vi "Parse Response.vi"(5 "Headers":string, 11 "error in (no error)":errorcluster) -> (6 "Response code":u16, 8 "Parsed headers":variant, 15 "error out":errorcluster)   [LabVIEW 2023, in "Weather Request Loop.lvlib"]
doc: "Parses the header block from an HTTP response. Returns the response code and a variant containing the parsed headers. The variant contains an attribute for each header, with the name of each attribute corresponding to the name of a header, converted to lower case. The value of each attribute is the value of that corresponding header."
uses:
  Weather Request Loop.lvlib
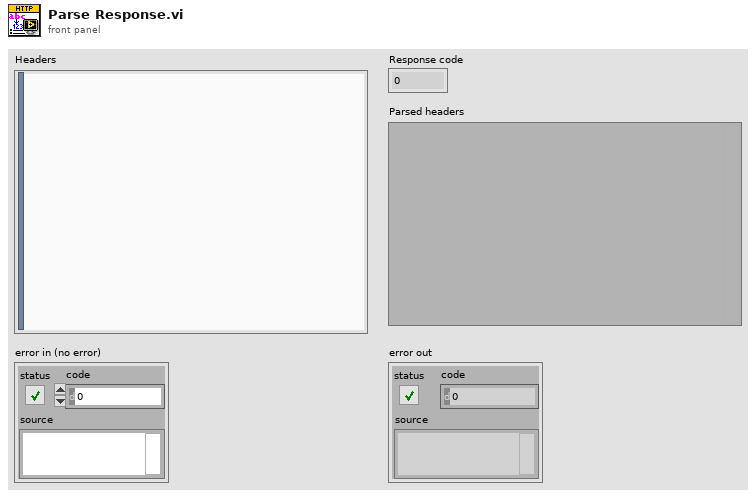
[diagram p1: front panel]
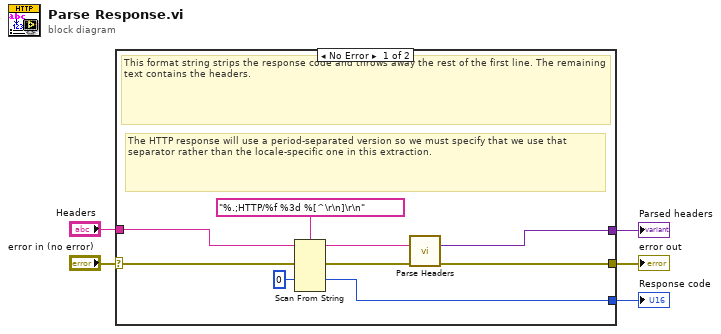
[diagram p0: block diagram]
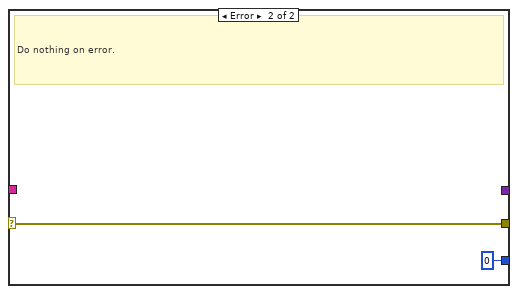
[diagram p2: hidden frame]
diagram:
  n1 = case shown="No Error" "error in (no error)" {
    selector: "error in (no error)" -> [w11 w16]
    tunnel: "Headers" -> [w14 _]
    tunnel: [w10 _] -> w5
    tunnel: [w12 w16] -> w4
    tunnel: [w8 u16 0] -> w3
    frame No Error {
      # "The HTTP response will use a period-separated version so we must specify that we use that separator rather than the locale-specific one in this extraction."
      # "This format string strips the response code and throws away the rest of the first line. The remaining text contains the headers."
      n2 = Scan From String(format string="%.;HTTP/%f %3d %[^\r\n]\r\n" ("regular expression"), input string=w14, error in=w11, default 2=u16 0 ("default value 2")) -> (remaining string=w6:string, error out=w13:errorcluster, output 2=w8:u16)  [unwired: 5 in, 1 out]
      n3 = call "Parse Headers.vi"("Headers"=w6, "error in (no error)"=w13) -> ("Parsed headers"=w10:variant, "error out"=w12:errorcluster)  [unwired: 12 in]
    }
    frame Error {
      # "Do nothing on error."
    }
  }
  "error out" <- w4
  "Response code" <- w3
  "Parsed headers" <- w5
